vi "Counter_reset.vi"(9 "reset":bool, 10 "enable":bool=TRUE, 11 "limit":u16) -> (2 "count = limit?":bool, 3 "count":u16)   [LabVIEW 2017]
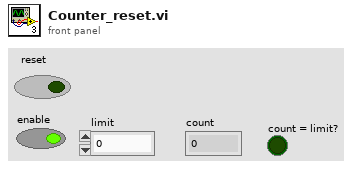
[diagram p1: front panel]
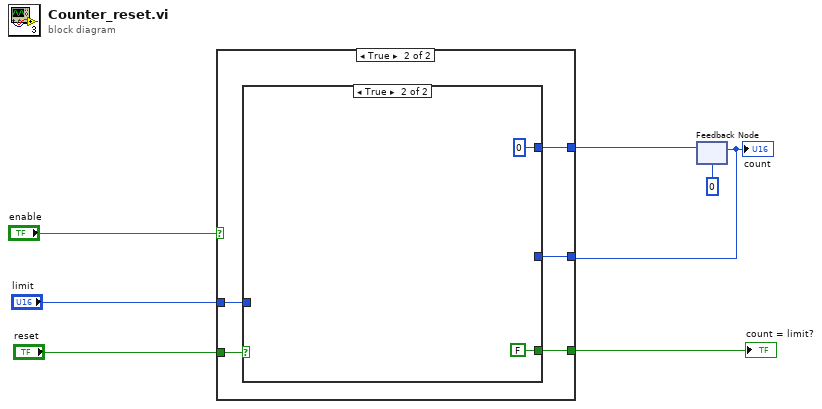
[diagram p0: block diagram]
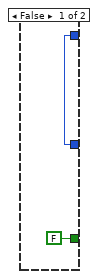
[diagram p2: hidden frame]
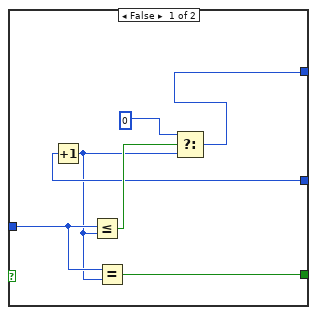
[diagram p3: hidden frame]
diagram:
  n1 = feedback #1(u16 0) -> (w4:u16)
  "count" <- w4
  n2 = case shown="True" "enable" {
    tunnel: "limit" -> [_ w14]
    tunnel: [w9 w13] -> w5
    tunnel: w4 -> [w9 w11]
    tunnel: "reset" -> [_ w12]
    tunnel: [FALSE w10] -> w1
    frame False {
    }
    frame True {
      n3 = case shown="True" w12 {
        tunnel: w14 -> [w17 _]
        tunnel: [w18 u16 0] -> w13
        tunnel: w11 -> [w19 _]
        tunnel: [w15 FALSE] -> w10
        frame False {
          n4 = Increment(x=w19) -> (x+1=w16:u16)
          n5 = Less Or Equal?(x=w17, y=w16) -> (x <= y?=w20:bool)
          n6 = Equal?(x=w17, y=w16) -> (x = y?=w15:bool)
          n7 = Select(t=u16 0, s=w20, f=w16) -> (s? t:f=w18:u16)
        }
        frame True {
        }
      }
    }
  }
  "count = limit?" <- w1
  n8 = feedback-in #1(w5) -> ()
